vi "Write LNA Active.vi"(8 "error in (no error)":errorcluster, 10 "LNA Active?":bool, 11 "Client Controller in":refnum<class "Client Controller.lvclass">) -> (0 "error out":errorcluster, 3 "Client Controller out":refnum<class "Client Controller.lvclass">)   [LabVIEW 2026, in "Client Controller.lvlib" / "Client Controller.lvclass"]
uses:
  Client Controller.lvclass
  Client Controller.lvclass/Client Controller.ctl
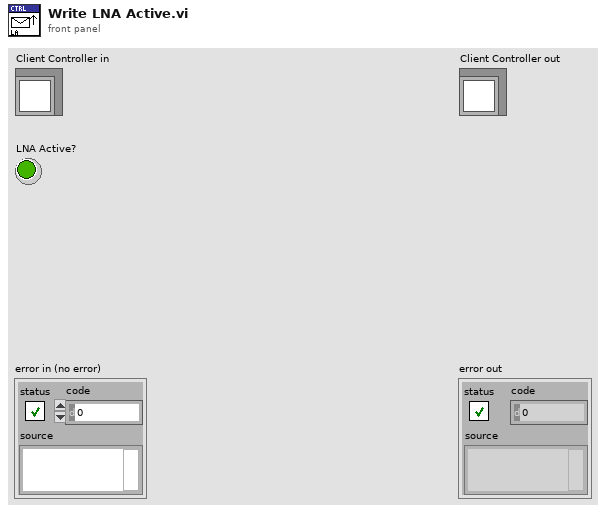
[diagram p1: front panel]
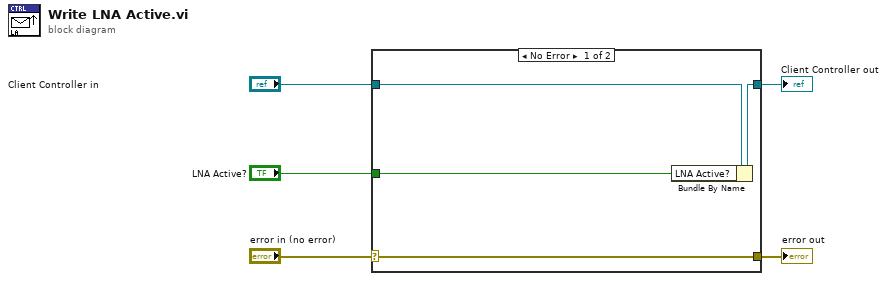
[diagram p0: block diagram]
diagram:
  n1 = case shown="No Error" "error in (no error)" {
    selector: "error in (no error)" -> [w9 w10]
    tunnel: [w9 w10] -> w4
    tunnel: [w7 w11] -> w2
    tunnel: "Client Controller in" -> [w8 w11]
    tunnel: "LNA Active?" -> [w6 _]
    frame No Error {
      n2 = Bundle By Name(cluster=w8, "LNA Active?"=w6) -> (w7:refnum<class "Client Controller.lvclass">)
    }
    frame Error {
    }
  }
  "error out" <- w4
  "Client Controller out" <- w2
